vi "pb_error_handler.vi"(8 "error in (no error)":errorcluster, 10 "return code":i32, 11 "path in":path=path "C:/Program Files/SpinCore/SpinAPI/dll/spinapi.dll") -> (0 "error out":errorcluster, 3 "path out":path)   [LabVIEW 2018]
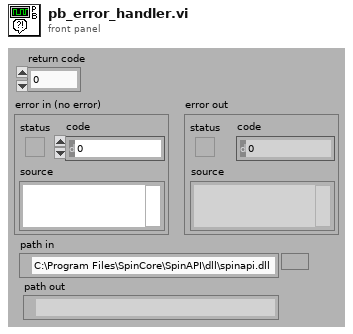
[diagram p1: front panel]
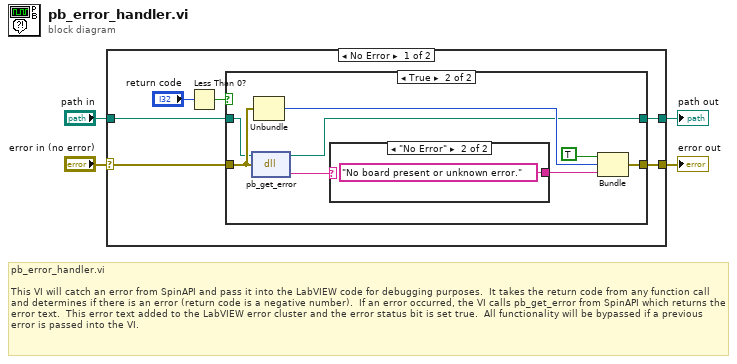
[diagram p0: block diagram]
diagram:
  # "pb_error_handler.vi\n\nThis VI will catch an error from SpinAPI and pass it into the LabVIEW code for debugging purposes.  It takes the return code from any function call and determines if there is an error (return code is a negative number).  If an error occurred, the VI calls pb_get_error from SpinAPI which returns the error text.  This error text added to the LabVIEW error cluster and the error status bit is set true.  All functionality will be bypassed if a previous error is passed into the VI."
  n1 = case shown="No Error" "error in (no error)" {
    selector: "error in (no error)" -> [w8 w24]
    tunnel: [w7 w24] -> w3
    tunnel: "path in" -> [w6 w23]
    tunnel: [w5 w23] -> w1
    frame No Error {
      n2 = Less Than 0?(x="return code") -> (x < 0?=w9:bool)
      n3 = case shown="True" w9 {
        tunnel: w8 -> [w12 w18]
        tunnel: [w12 w17] -> w7
        tunnel: w6 -> [w11 w14]
        tunnel: [w11 w13] -> w5
        frame False {
        }
        frame True {
          n4 = dll-call lib="C:/Program Files/SpinCore/SpinAPI/dll/spinapi.dll" fn="pb_get_error"(path in=w14, error in=w18) -> (path out=w13:path, "return type"=w16:string)  [unwired: 1 in, 1 out]
          n5 = Unbundle(w18) -> ("code"=w19:i32)  [unwired: 2 out]
          n6 = case shown="\"No Error\"" w16 {
            selector: w16 -> [w21 _]
            tunnel: [w21 "No board present or unknown error."] -> w15
            frame Default {
            }
            frame "No Error" {
            }
          }
          n7 = Bundle(TRUE, "code"=w19, w15) -> (w17:cluster{bool, "code":i32, string})  [unwired: 1 out]
        }
      }
    }
    frame Error {
    }
  }
  "error out" <- w3
  "path out" <- w1
